vi "Top Level VI Reference.vi"() -> ()   [LabVIEW 2011]
panel:
  in  "Path to Root Directory":path
  in  "This VI":refnum<vi>
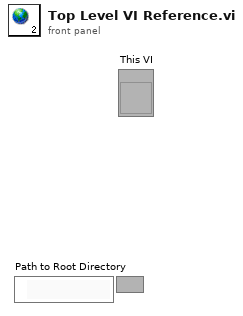
[diagram p1: front panel]
diagram:
